vi "Send Receive (SubVI).vi"(8 "error in (no error)":errorcluster, 10 "Command":string="?", 11 "VISA Refnum in":refnum<visa-resource-name>) -> (0 "error out":errorcluster, 2 "Response":string, 3 "VISA Refnum out":refnum<visa-resource-name>)   [LabVIEW 2015]
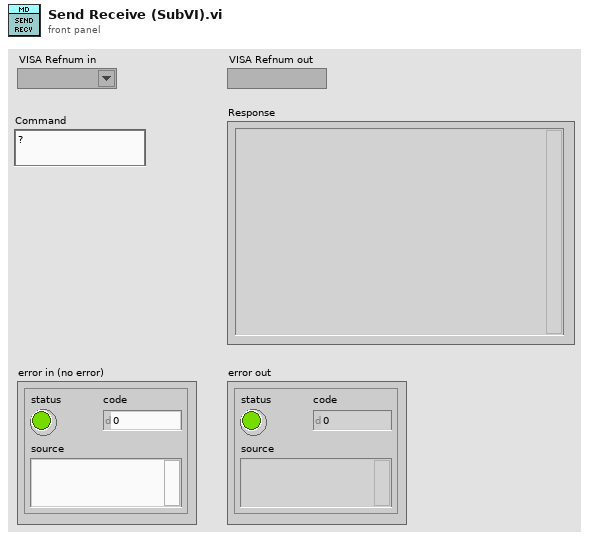
[diagram p1: front panel]
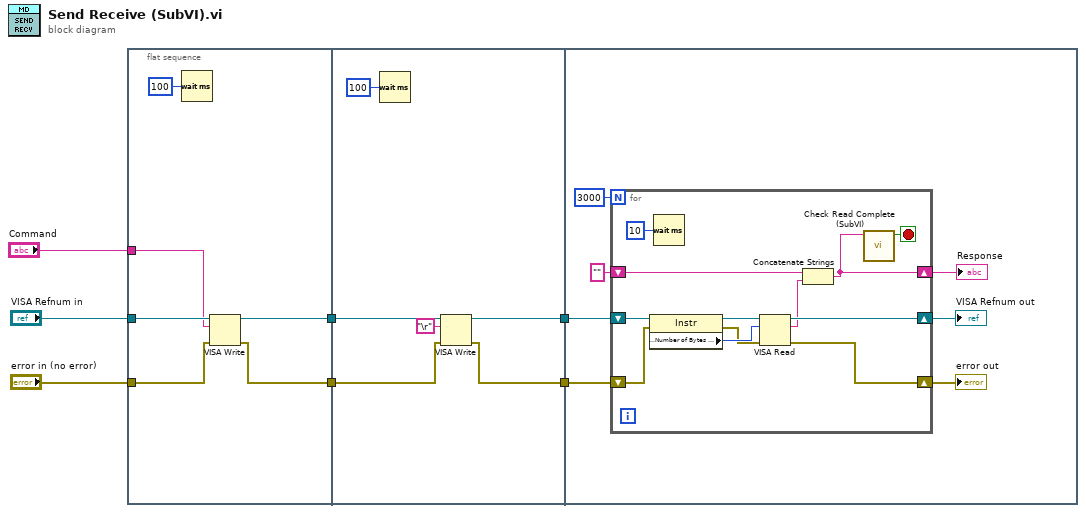
[diagram p0: block diagram]
diagram:
  n1 = flat-sequence {
    tunnel: "VISA Refnum in" -> [w12]
    tunnel: "error in (no error)" -> [w10]
    tunnel: [w9] -> w3
    tunnel: [w11] -> w2
    tunnel: "Command" -> [w8]
    tunnel: [w14] -> w5
    tunnel: [w16] -> w4
    tunnel: w3 -> [w15]
    tunnel: w2 -> [w17]
    tunnel: w5 -> [w26]
    tunnel: w4 -> [w25]
    frame #0 {
      n2 = Wait (ms)(milliseconds to wait=u32 100) -> ()  [unwired: 1 out]
      n3 = VISA Write(VISA resource name=w12, write buffer=w8, error in (no error)=w10) -> (VISA resource name out=w11:refnum<visa-resource-name>, error out=w9:errorcluster)  [unwired: 1 out]
    }
    frame #1 {
      n4 = Wait (ms)(milliseconds to wait=u32 100) -> ()  [unwired: 1 out]
      n5 = VISA Write(VISA resource name=w17, write buffer="\r", error in (no error)=w15) -> (VISA resource name out=w16:refnum<visa-resource-name>, error out=w14:errorcluster)  [unwired: 1 out]
    }
    frame #2 {
      n6 = for {
        N: 3000 -> [_]
        shift-right: [w38] -> w23
        shift-left: w25 -> [w36]
        shift-right: [w37] -> w24
        shift-left: w26 -> [w30]
        shift-right: [w27] -> w20
        shift-left: "" -> [w32]
        stop <- w28 stop-if-true
        n7 = property class="Instr"(reference=w36, error in=w30) -> (reference out=w34:refnum<visa-resource-name>, error out=w29:errorcluster, "Serial Settings:Number of Bytes at Serial Port"=w33:u32)
        n8 = Wait (ms)(milliseconds to wait=u32 10) -> ()  [unwired: 1 out]
        n9 = VISA Read(VISA resource name=w34, byte count=w33, error in (no error)=w29) -> (VISA resource name out=w38:refnum<visa-resource-name>, read buffer=w35:string, error out=w37:errorcluster)  [unwired: 1 out]
        n10 = Concatenate Strings(w32, w35) -> (w27:string)
        n11 = call "Check Read Complete (SubVI).vi"("JSON String"=w27) -> ("Complete?"=w28:bool)  [unwired: 10 in]
      }
      "error out" <- w24
      "VISA Refnum out" <- w23
      "Response" <- w20
    }
  }
